vi "Save Sensor.vi"(8 "error in (no error)":errorcluster, 11 "Edit Sensor Model in":refnum<class "Edit Sensor Model.lvclass">) -> (0 "error out":errorcluster, 3 "Edit Sensor Model out":refnum<class "Edit Sensor Model.lvclass">)   [LabVIEW 2013, in "Edit Sensor Model.lvlib" / "Edit Sensor Model.lvclass"]
uses:
  Edit Sensor Model.lvclass
  Edit Sensor Model.lvclass/Edit Sensor Model.ctl
  Common/File IO/File IO.lvlib
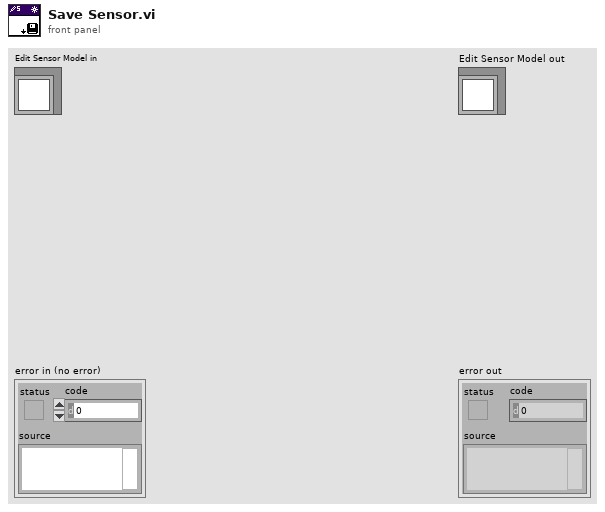
[diagram p1: front panel]
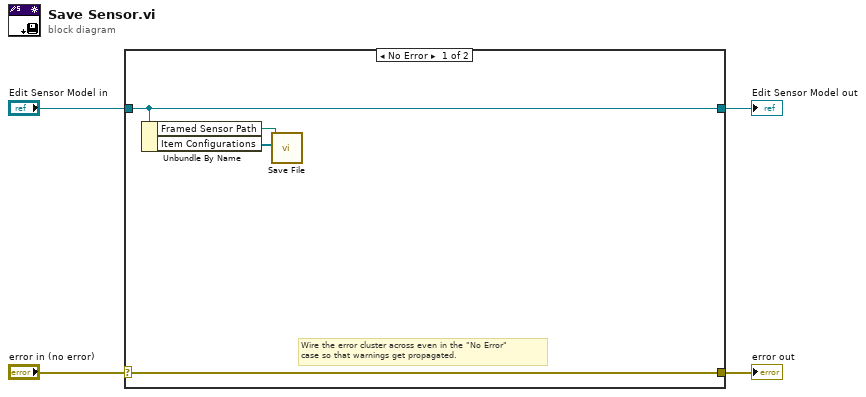
[diagram p0: block diagram]
diagram:
  n1 = case shown="No Error" "error in (no error)" {
    selector: "error in (no error)" -> [w8 w10]
    tunnel: [w8 w10] -> w2
    tunnel: [w6 w9] -> w3
    tunnel: "Edit Sensor Model in" -> [w6 w9]
    frame No Error {
      # "Wire the error cluster across even in the \"No Error\"\ncase so that warnings get propagated."
      n2 = Unbundle By Name(w6) -> ("Framed Sensor Path"=w5:path, "Item Configurations"=w7:refnum<class "Item Configuration.lvclass">[])
      n3 = call "Save File.vi"("Item Configurations"=w7, "File Path"=w5) -> ()  [unwired: 9 in, 1 out]
    }
    frame Error {
    }
  }
  "error out" <- w2
  "Edit Sensor Model out" <- w3
